vi "Portcullis_Brain.vi"(3 "Portcullis Enable":bool) -> (0 "Portcullis Active":bool, 1 "Intake_Pos":T2, 2 "Arm_Defense":T1)   [LabVIEW 2015]
uses:
  Intake Enum..ctl
  Arm_defense_Type_Def.ctl
  Portcullis_type_def.ctl
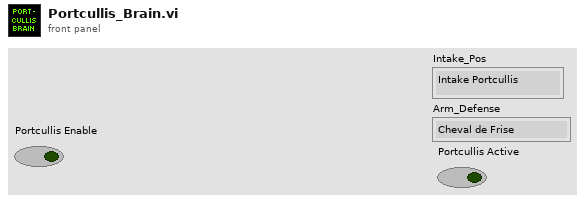
[diagram p1: front panel]
types:
  T1 = typedef "Arm_defense_Type_Def.ctl" = enum16{"Cheval de Frise", "Portcullis", "Ball_Pickup"}
  T2 = typedef "Intake Enum..ctl" = enum16{"Intake Portcullis", "Intake Ball Pickup", "Intake Cheval", " Intake Raised"}
  T3 = typedef "Portcullis_type_def.ctl" = enum16{"Lower", "Off"}
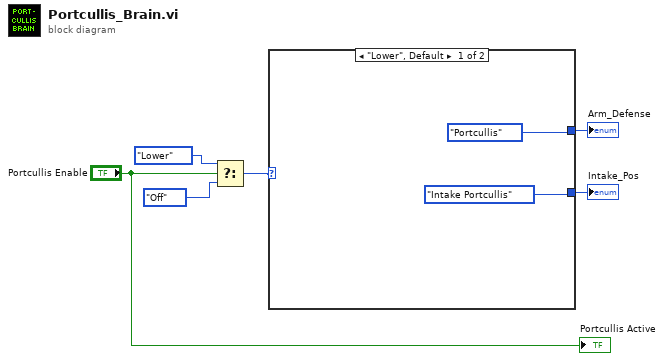
[diagram p0: block diagram]
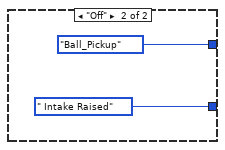
[diagram p2: hidden frame]
diagram:
  n1 = Select(t=Portcullis_type_def."Lower", s="Portcullis Enable", f=Portcullis_type_def."Off") -> (s? t:f=w6:T3)
  n2 = case shown="\"Lower\", Default" w6 {
    tunnel: [Arm_defense_Type_Def."Portcullis" ("P1_Value") Arm_defense_Type_Def."Ball_Pickup" ("P1_Value")] -> w1
    tunnel: [Intake_Enum.."Intake Portcullis" ("P1_Value") Intake_Enum.." Intake Raised" ("P1_Value")] -> w2
    frame "Lower", Default {
    }
    frame "Off" {
    }
  }
  "Intake_Pos" <- w2
  "Arm_Defense" <- w1
  "Portcullis Active" <- "Portcullis Enable"
